vi "XY Graph Check X Arrays Compatibility.vi"(6 "epsilon (machine)":dbl=2.220446049250313e-16, 8 "Existing Y Array":dbl[](array[numeric]), 9 "Existing X Array in":dbl[](array[numeric]), 11 "New X Array in":dbl[](array[numeric])) -> (0 "Y Array out":dbl[](array[numeric]), 1 "X Array out":dbl[](array[numeric]), 3 "Compatible Arrays?":bool)   [LabVIEW 2021, in "XY Graph Add-Ons.lvlib"]
uses:
  XY Graph Add-Ons.lvlib
  Arrays/Arrays.lvlib
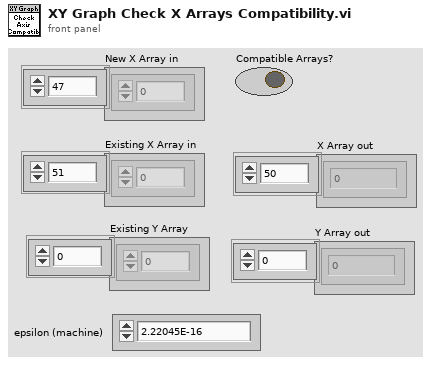
[diagram p1: front panel]
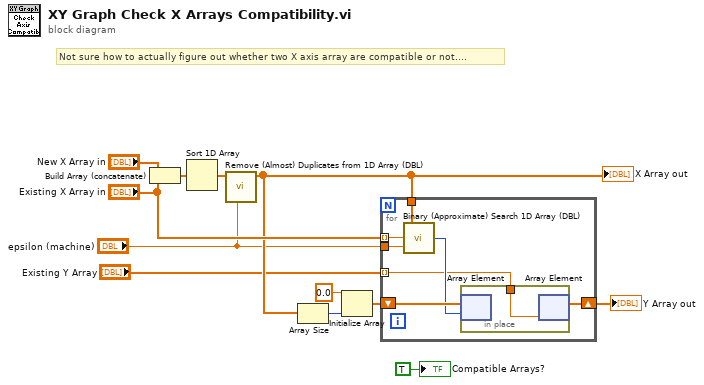
[diagram p0: block diagram]
diagram:
  # "Not sure how to actually figure out whether two X axis array are compatible or not...."
  n1 = Build Array (concatenate)("New X Array in", "Existing X Array in") -> (w11:dbl[])
  n2 = Sort 1D Array(array=w11) -> (sorted array=w1:dbl[])
  n3 = call "Remove (Almost) Duplicates from 1D Array (DBL).vi"("epsilon (machine)"="epsilon (machine)", "Input Array"=w1) -> ("Output Array"=w8:dbl[])  [unwired: 8 in, 1 out]
  "X Array out" <- w8
  n4 = Array Size(array=w8) -> (size(s)=w7:i32)
  n5 = Initialize Array(0.0 ("element"), w7) -> (w5:dbl[])
  n6 = for {
    tunnel: "Existing X Array in" -> [w19] mode=indexing
    tunnel: w8 -> [w18]
    shift-right: [w16] -> w4
    shift-left: w5 -> [w17]
    tunnel: "Existing Y Array" -> [w14] mode=indexing
    tunnel: "epsilon (machine)" -> [w13]
    n7 = call "Binary (Approximate) Search 1D Array (DBL).vi"("epsilon (machine)"=w13, "element"=w19, "1D array"=w18) -> ("index"=w15:i32)
    n8 = in-place {
      in-place-border: w14 -> [w20]
      n9 = in-place-array #1(w17, w15) -> ()  [unwired: 1 out]
      n10 = in-place-array #1(w20) -> (w16:dbl[])  [unwired: 1 out]
    }
  }
  "Y Array out" <- w4
  "Compatible Arrays?" <- TRUE ("Compatible Arrays?")
